vi "Search JSON.vi"(8 "error in":errorcluster, 10 "Name Array 2":string[](array[string]), 11 "Response body":string) -> (0 "error out":errorcluster, 3 "LabVIEW Text":string)   [LabVIEW 2024, in "GUI.lvlib"]
uses:
  GUI.lvlib
  <vilib>/addons/JSON API/JSON Value/Set from JSON string.vi
  <vilib>/addons/JSON API/JSON Scalar/Get as Text.vi
  <vilib>/addons/JSON API/JSON Value/JSON Value.lvclass
  <vilib>/addons/JSON API/Get Polymorphic/JSON GetSet.lvlib
  <vilib>/addons/JSON API/JSON Scalar/JSON Scalar.lvclass
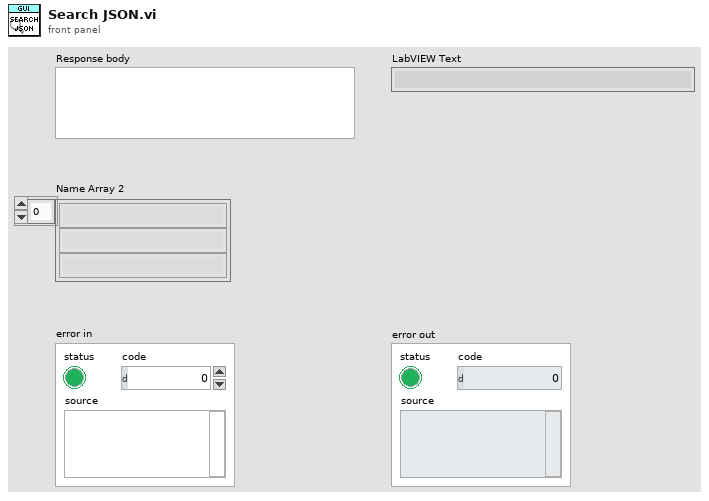
[diagram p1: front panel]
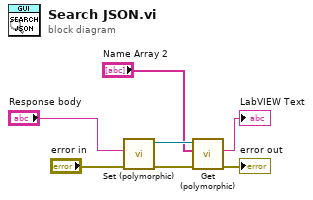
[diagram p0: block diagram]
diagram:
  n1 = call-poly <vilib>:"Set (polymorphic).vi"("error in (no error)"="error in", "JSON stream"="Response body") -> ("error out"=w5:errorcluster, "JSON Value out"=w6:refnum<class "JSON Value.lvclass">)  [unwired: 7 in, 1 out]
  n2 = call-poly <vilib>:"Get (polymorphic).vi"("error in (no error)"=w5, "Name Array"="Name Array 2", "JSON Scalar in"=w6) -> ("error out"=→"error out":errorcluster, "LabVIEW Text"=→"LabVIEW Text":string)  [unwired: 6 in, 1 out]
